vi "writeablock.vi"(8 "error in (no error)":errorcluster, 9 "BlockSize":i32, 10 "Array":dbl[][](array[numeric]), 11 "QuadraturePositionDecoder in":refnum<class "QuadraturePositionDecoder.lvclass">) -> (0 "error out":errorcluster, 3 "QuadraturePositionDecoder out":refnum<class "QuadraturePositionDecoder.lvclass">)   [LabVIEW 2014, in "QuadraturePositionDecoder.lvclass"]
uses:
  QuadraturePositionDecoder.lvclass
  private/HDF5Tools32/LabView/HDF5Tools.lvlib
  private/HDF5Tools32/LabView/Append To Dataset 2D Double.vi
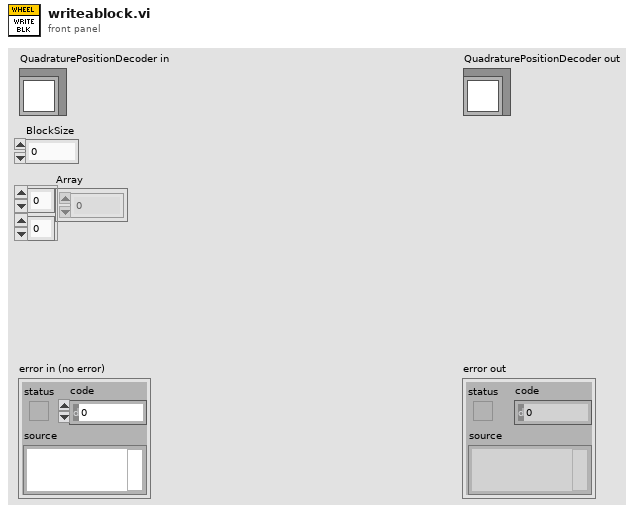
[diagram p1: front panel]
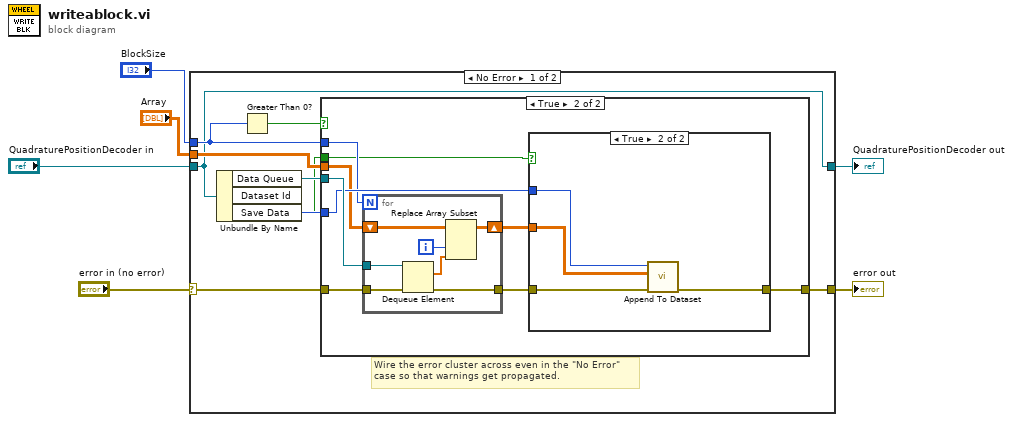
[diagram p0: block diagram]
diagram:
  n1 = case shown="No Error" "error in (no error)" {
    selector: "error in (no error)" -> [w11 w39]
    tunnel: [w10 w39] -> w5
    tunnel: [w8 w38] -> w3
    tunnel: "QuadraturePositionDecoder in" -> [w8 w38]
    tunnel: "BlockSize" -> [w13 _]
    tunnel: "Array" -> [w9 _]
    frame No Error {
      # "Wire the error cluster across even in the \"No Error\"\ncase so that warnings get propagated."
      n2 = Unbundle By Name(w8) -> ("Data Queue"=w15:refnum<queue>, "Dataset Id"=w12:i32, "Save Data"=w7:bool)
      n3 = Greater Than 0?(x=w13) -> (x > 0?=w14:bool)
      n4 = case shown="True" w14 {
        tunnel: w11 -> [w16 w24]
        tunnel: [w16 w22] -> w10
        tunnel: w13 -> [_ w19]
        tunnel: w15 -> [_ w25]
        tunnel: w12 -> [_ w21]
        tunnel: w9 -> [_ w18]
        tunnel: w7 -> [_ w17]
        frame False {
        }
        frame True {
          n5 = for {
            N: w19 -> [_]
            tunnel: w25 -> [w37]
            tunnel: w24 -> [w36]
            tunnel: [w35] -> w23
            shift-right: [w33] -> w20
            shift-left: w18 -> [w34]
            i -> [w32]
            n6 = Dequeue Element(queue=w37, error in (no error)=w36) -> (element=w31:dbl[], error out=w35:errorcluster)  [unwired: 1 in, 2 out]
            n7 = Replace Array Subset(array=w34, new element=w31, index (col)=w32) -> (w33:dbl[][])  [unwired: 1 in]
          }
          n8 = case shown="True" w17 {
            tunnel: w20 -> [_ w30]
            tunnel: w23 -> [w26 w29]
            tunnel: [w26 w28] -> w22
            tunnel: w21 -> [_ w27]
            frame False {
            }
            frame True {
              n9 = call-poly "Append To Dataset.vi"("Error in (no error)"=w29, "Data"=w30, "Dataset id in"=w27) -> ("Error out"=w28:errorcluster)  [unwired: 7 in, 1 out]
            }
          }
        }
      }
    }
    frame Error {
    }
  }
  "error out" <- w5
  "QuadraturePositionDecoder out" <- w3
